vi "main_FC.vi"() -> ()   [LabVIEW 2017]
uses:
  <vilib>/addons/control/pid/pid.llb/PID (DBL).vi
  <vilib>/addons/control/pid/NI_PID_pid.lvlib
panel:
  in  "Tab Control":enum32{"Page 1", "Page 2"}(tab)
  in  "Menu Ring":u16(ring) items=["OFF", "Automatic", "Manual"]
  out "Waveform Chart":T1(graph) caption="Response Chart"
  in  "Mode":bool=TRUE
  in  "Pause Button":bool
  in  "Reset Chart":bool
  in  "Save as Excel":bool
  in  "Save as image":bool
  in  "Block Diagram":bool
  out "FR":dbl
  out "Control Action":dbl
  in  "Flow rate setpoint":dbl=25.0
  in  "Pump":bool=TRUE
  in  "ON/OFF":bool
  in  "Exit":bool
  in  "PID gains":cluster{"Kp":dbl, "KI":dbl, "Kd":dbl}={"Kp"=1.0, "KI"=0.0, "Kd"=0.0}
  out "NI1":tag caption="NI device"
  in  "Main board":bool
  # "Flow Control Training System"
  # "Flow sensor Reading"
  # "Block Diagram of \nthe Flow rate Closed-loop Control System"
  # "Automatic Mode"
  # "ON/OFF"
  # "Automatic mode"
  # "Actuator ON/OFF"
  # "desired FR"
  # "Controller\n(PID)"
  # "Actuator\n(Pump)"
  # "System"
  # "Head (d_Pressure)"
  # "error signal"
  # "+"
  # "-"
  # "Control Action\n(0% - 100%)"
  # "actual FR"
  # "Flow rate sensor"
  # "Block Diagram of \nthe Flow rate Open-loop Control System"
  # "Manual Mode"
  # "ON/OFF"
  # "Manual mode"
  # "Actuator ON/OFF"
  # "Actuator\n(Pump)"
  # "Head (d_Pressure)"
  # "System"
  # "Signal\nConditioner"
  # "Angle"
  # "Potentiometer"
  # "Control Action\n(0% - 100%)"
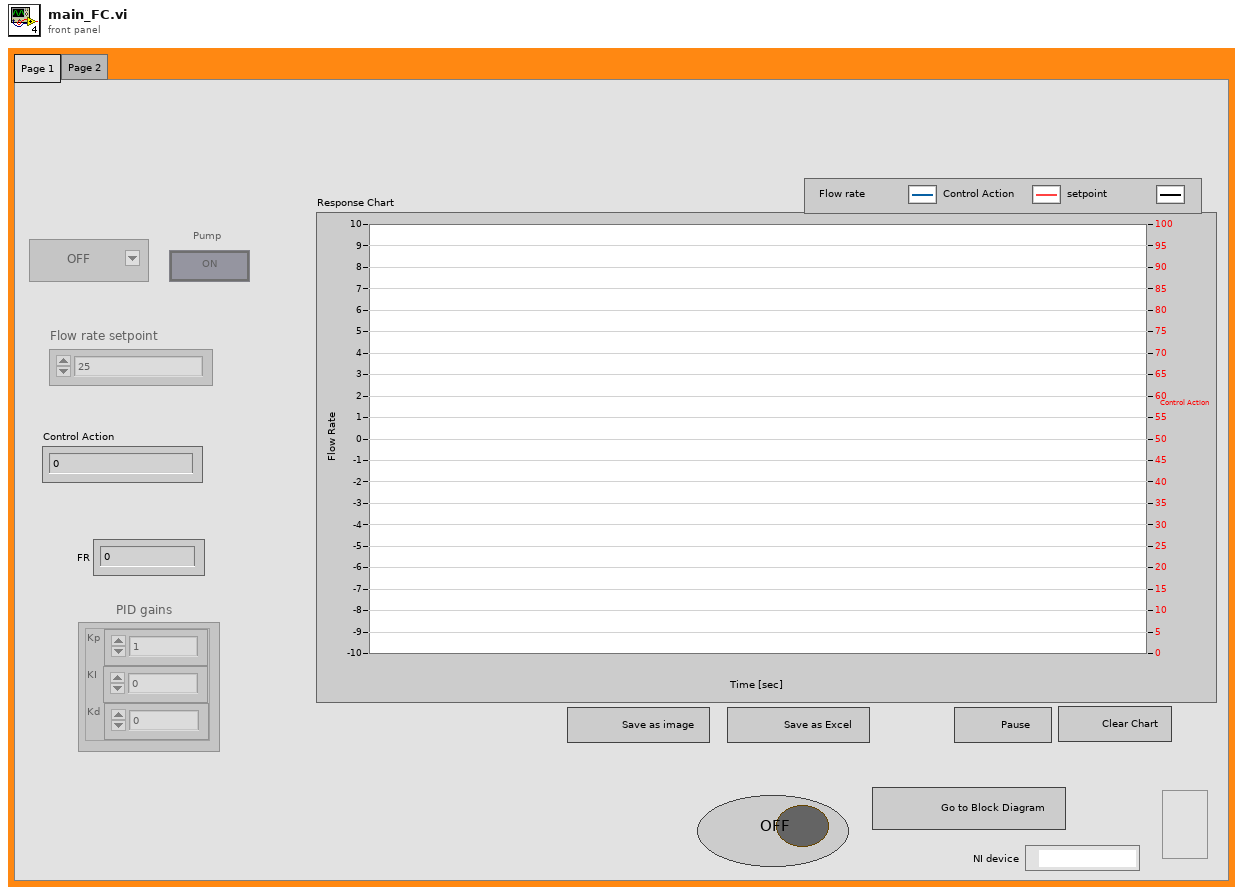
[diagram p1: front panel]
types:
  T1 = cluster{"Scalar":dbl, "f":dbl, "Flow rate setpoint":dbl}
  T2 = enum32{"Invalid", "Standard", "Closed", "Hidden", "Minimized", "Maximized"}
  T3 = enum8{"Enabled", "Disabled", "Disabled and Grayed Out"}
  T4 = cluster{"Scalar":dbl, "f":dbl, "Flow rate setpoint":dbl}[]
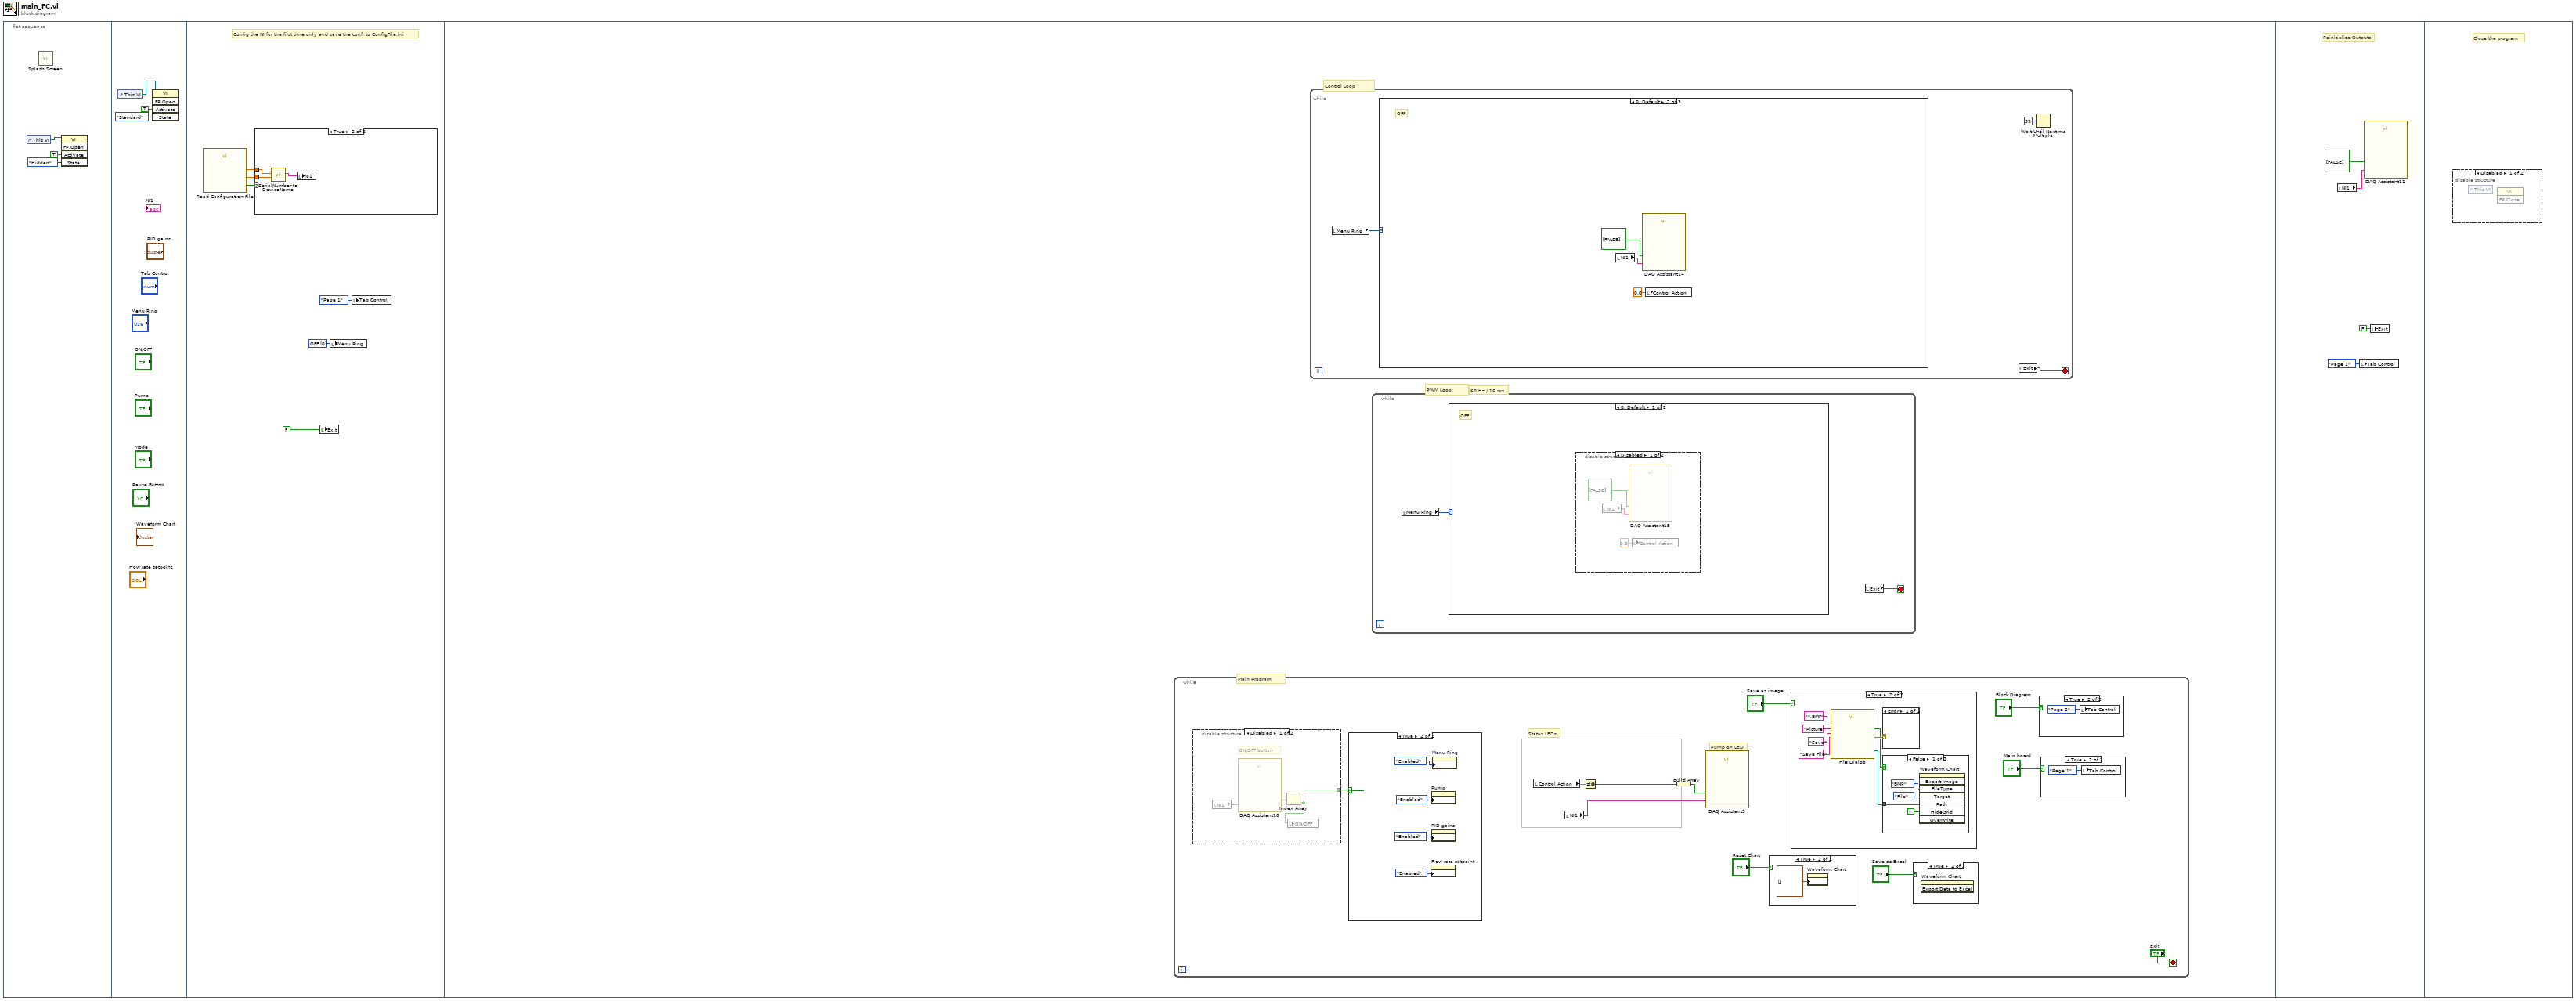
[diagram p0: block diagram]
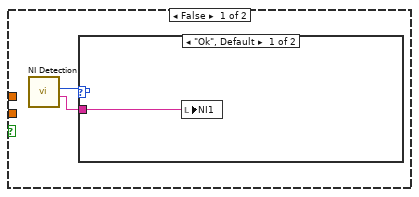
[diagram p2: hidden frame]
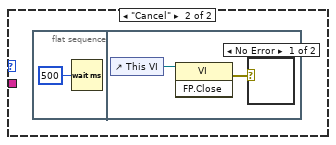
[diagram p3: hidden frame]
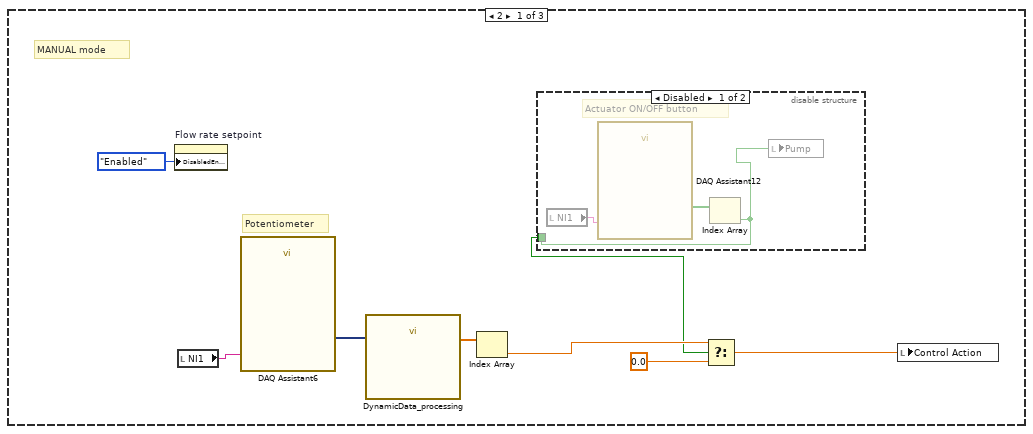
[diagram p5: hidden frame]
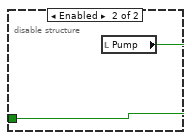
[diagram p6: hidden frame]
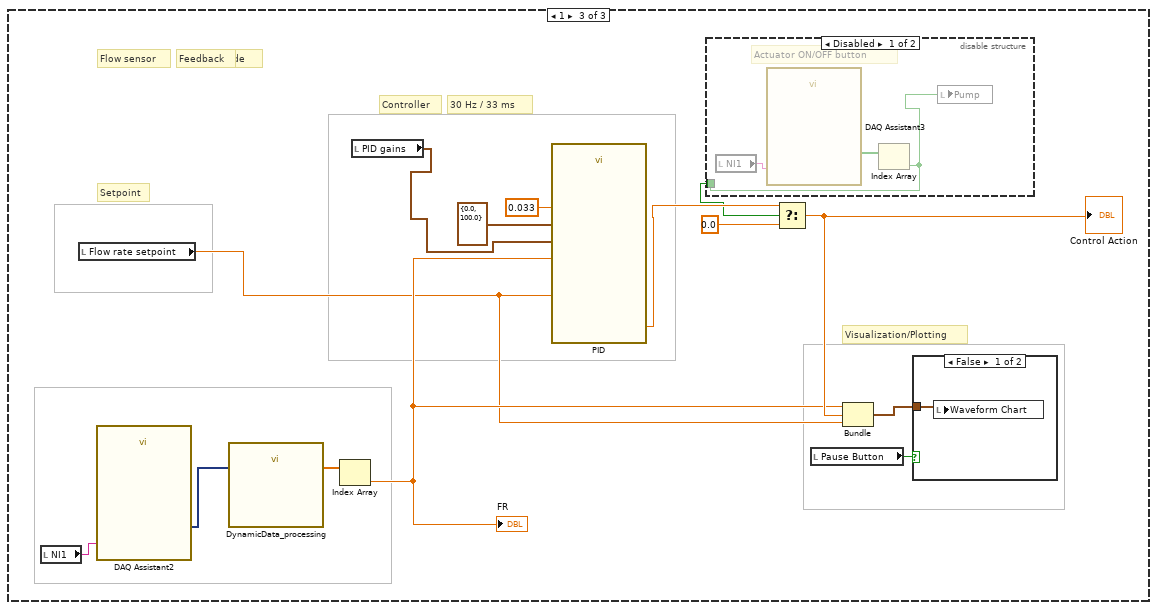
[diagram p7: hidden frame]
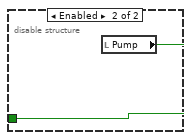
[diagram p8: hidden frame]
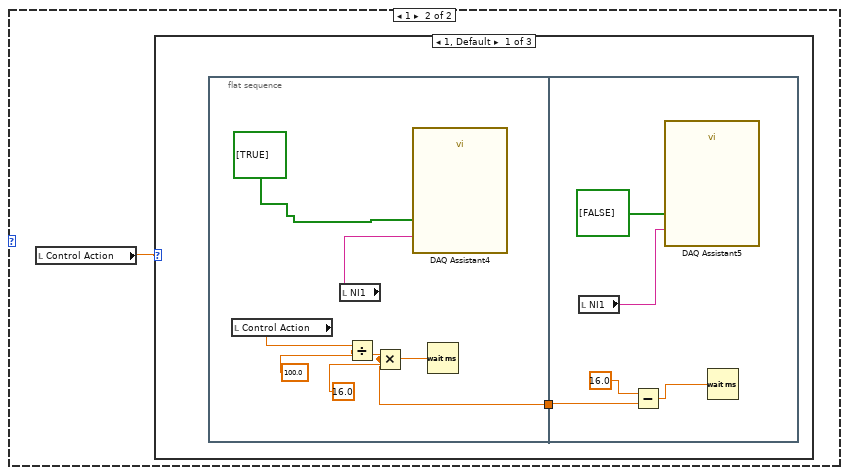
[diagram p11: hidden frame]
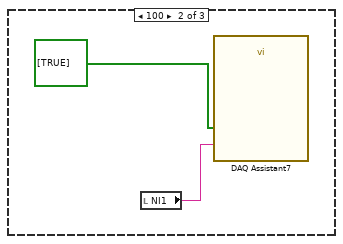
[diagram p12: hidden frame]
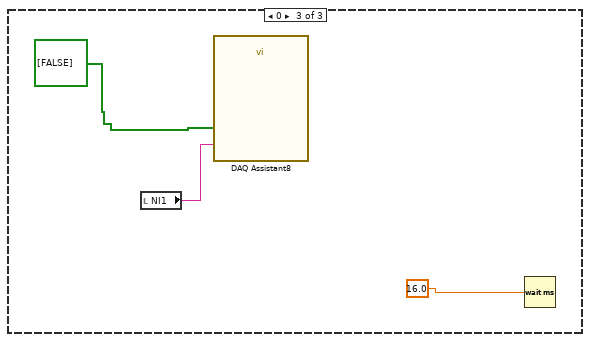
[diagram p13: hidden frame]
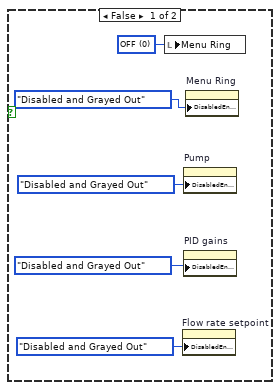
[diagram p14: hidden frame]
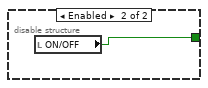
[diagram p15: hidden frame]
diagram:
  n1 = flat-sequence {
    frame #0 {
      n2 = control-ref of="This VI"() -> (w3:refnum<vi>)
      n3 = call "Splash Screen.vi"() -> ()  [unwired: 11 in, 1 out]
      n4 = invoke class="VI" method="FP.Open"(reference=w3, "Activate"=TRUE ("Activate?"), "State"=T2."Hidden") -> ()  [unwired: 2 in, 5 out]
    }
    frame #1 {
      n5 = control-ref of="This VI"() -> (w4:refnum<vi>)
      n6 = invoke class="VI" method="FP.Open"(reference=w4, "Activate"=TRUE ("Activate?"), "State"=T2."Standard") -> ()  [unwired: 2 in, 5 out]
    }
    frame #2 {
      w7 = u16 0 items=["OFF", "Automatic", "Manual"] ("Menu Ring")
      # "Config the NI for the first time only and save the conf. to ConfigFile.ini"
      n7 = call "Read Configuration File.vi"() -> ("Serial Numbers Found"=w10:bool, "NI1"=w11:dbl, "NI2"=w12:dbl)  [unwired: 13 in]
      n8 = case shown="True" w10 {
        tunnel: w11 -> [_ w21]
        tunnel: w12 -> [_ w20]
        frame False {
          n9 = call "NI Detection.vi"() -> ("NI 1"=w13:tag, "Ok/Cancel"=w14:enum16{"Ok", "Cancel"})  [unwired: 8 in, 1 out]
          n10 = case shown="\"Ok\", Default" w14 {
            tunnel: w13 -> [w15 _]
            frame "Ok", Default {
              n11 = local write "NI1"(w15) -> ()
            }
            frame "Cancel" {
              n12 = flat-sequence {
                frame #0 {
                  n13 = Wait (ms)(milliseconds to wait=u32 500) -> ()  [unwired: 1 out]
                }
                frame #1 {
                  n14 = control-ref of="This VI"() -> (w18:refnum<vi>)
                  n15 = invoke class="VI" method="FP.Close"(reference=w18) -> (error out=w17:errorcluster)  [unwired: 2 in, 2 out]
                  n16 = case shown="No Error" w17 {
                    frame No Error {
                    }
                    frame Error {
                    }
                  }
                }
              }
            }
          }
        }
        frame True {
          n17 = call "SerialNumber to DeviceName.vi"("NI2 Serial Number"=w20, "NI1 Serial Number"=w21) -> ("NI1 Device Name"=w19:tag)  [unwired: 8 in, 1 out]
          n18 = local write "NI1"(w19) -> ()
        }
      }
      n19 = local write "Exit"(FALSE ("ON / OFF program")) -> ()
      n20 = local write "Menu Ring"(w7) -> ()
      n21 = local write "Tab Control"(enum32{"Page 1", "Page 2"}."Page 1" ("Tab Control")) -> ()
    }
    frame #3 {
      # "Control Loop"
      # "60 Hz / 16 ms"
      # "PWM Loop"
      # "Main Program"
      n22 = while {
        stop <- "Exit" stop-if-true
        # "Pump on LED"
        # "Status LEDs"
        n23 = disable-structure shown="Disabled" {
          disable-tunnel: [w103 w106] -> w83
          frame Disabled {
            # "ON/OFF button"
            n24 = local read "NI1"() -> (w105:tag)
            n25 = call "DAQ Assistant10"("device name"=w105) -> ("data"=w104:bool[])  [unwired: 16 in, 2 out]
            n26 = Index Array(array=w104) -> (element=w103:bool)  [unwired: 1 in]
            n27 = local write "ON/OFF"(w103) -> ()
          }
          frame Enabled {
            n28 = local read "ON/OFF"() -> (w106:bool)
          }
        }
        n29 = case shown="True" w83 {
          frame False {
            w98 = u16 0 items=["OFF", "Automatic", "Manual"] ("Menu Ring")
            n30 = local write "Menu Ring"(w98) -> ()
            n31 = property on="Flow rate setpoint" class="DigNum (strict)"("DisabledEnum"=T3."Disabled and Grayed Out" ("Disabled")) -> ()  [unwired: 2 in, 2 out]
            n32 = property on="Pump" class="Bool (strict)"("DisabledEnum"=T3."Disabled and Grayed Out" ("Disabled")) -> ()  [unwired: 2 in, 2 out]
            n33 = property on="PID gains" class="Clust (strict)"("DisabledEnum"=T3."Disabled and Grayed Out" ("Disabled")) -> ()  [unwired: 2 in, 2 out]
            n34 = property on="Menu Ring" class="Ring (strict)"("DisabledEnum"=T3."Disabled and Grayed Out" ("Disabled")) -> ()  [unwired: 2 in, 2 out]
          }
          frame True {
            n35 = property on="Flow rate setpoint" class="DigNum (strict)"("DisabledEnum"=T3."Enabled" ("Disabled")) -> ()  [unwired: 2 in, 2 out]
            n36 = property on="Pump" class="Bool (strict)"("DisabledEnum"=T3."Enabled" ("Disabled")) -> ()  [unwired: 2 in, 2 out]
            n37 = property on="PID gains" class="Clust (strict)"("DisabledEnum"=T3."Enabled" ("Disabled")) -> ()  [unwired: 2 in, 2 out]
            n38 = property on="Menu Ring" class="Ring (strict)"("DisabledEnum"=T3."Enabled" ("Disabled")) -> ()  [unwired: 2 in, 2 out]
          }
        }
        n39 = local read "Control Action"() -> (w86:dbl)
        n40 = local read "NI1"() -> (w85:tag)
        n41 = Not Equal To 0?(x=w86) -> (x != 0?=w87:bool)
        n42 = Build Array(w87) -> (w88:bool[])
        n43 = call "DAQ Assistant9"("data"=w88, "device name"=w85) -> ()  [unwired: 16 in, 2 out]
        n44 = case shown="True" "Reset Chart" {
          frame False {
          }
          frame True {
            n45 = property on="Waveform Chart" class="WFChart (strict)"("History Data"=T4 []) -> ()  [unwired: 2 in, 2 out]
          }
        }
        n46 = case shown="True" "Save as image" {
          frame False {
          }
          frame True {
            n47 = call "File Dialog"("prompt"="Save File", "button label"="Save", "pattern (all files)"="*.BMP", "pattern label"="Picture") -> ("selected path"=w108:path, "cancelled"=w107:bool, "error out"=w109:errorcluster)  [unwired: 8 in, 1 out]
            n48 = case shown="Error" w109 {
              frame No Error {
              }
              frame Error {
              }
            }
            n49 = case shown="False" w107 {
              tunnel: w108 -> [w115 _]
              frame False {
                n50 = invoke on="Waveform Chart" class="WFChart (strict)" method="Export Image"("FileType"=enum32{"BMP", "EPS", "EMF", "PICT"}."BMP" ("File Type"), "Target"=enum32{"File", "Clipboard"}."File", "Path"=w115, "HideGrid"=TRUE ("Hide Grid")) -> ()  [unwired: 4 in, 8 out]
              }
              frame True {
              }
            }
          }
        }
        n51 = case shown="True" "Save as Excel" {
          frame False {
          }
          frame True {
            n52 = invoke on="Waveform Chart" class="WFChart (strict)" method="Export Data to Excel"() -> ()  [unwired: 3 in, 3 out]
          }
        }
        n53 = case shown="True" "Block Diagram" {
          frame False {
          }
          frame True {
            n54 = local write "Tab Control"(enum32{"Page 1", "Page 2"}."Page 2" ("Tab Control")) -> ()
          }
        }
        n55 = case shown="True" "Main board" {
          frame False {
          }
          frame True {
            n56 = local write "Tab Control"(enum32{"Page 1", "Page 2"}."Page 1" ("Tab Control")) -> ()
          }
        }
      }
      n57 = while {
        stop <- w22 stop-if-true
        n58 = local read "Menu Ring"() -> (w23:u16)
        n59 = case shown="0, Default" w23 {
          frame 2 {
            # "MANUAL mode"
            # "Potentiometer"
            n60 = property on="Flow rate setpoint" class="DigNum (strict)"("DisabledEnum"=T3."Enabled" ("Disabled")) -> ()  [unwired: 2 in, 2 out]
            n61 = local read "NI1"() -> (w32:tag)
            n62 = call "DAQ Assistant6"("device name"=w32) -> ("data"=w30:dynamicdata)  [unwired: 16 in, 2 out]
            n63 = call "DynamicData_processing.vi"("data"=w30) -> ("DATA"=w31:dbl[])
            n64 = Index Array(array=w31) -> (element=w29:dbl)  [unwired: 1 in]
            n65 = disable-structure shown="Disabled" {
              disable-tunnel: [w34 w36] -> w27
              frame Disabled {
                # "Actuator ON/OFF button"
                n66 = local read "NI1"() -> (w33:tag)
                n67 = call "DAQ Assistant12"("device name"=w33) -> ("data"=w35:bool[])  [unwired: 16 in, 2 out]
                n68 = Index Array(array=w35) -> (element=w34:bool)  [unwired: 1 in]
                n69 = local write "Pump"(w34) -> ()
              }
              frame Enabled {
                n70 = local read "Pump"() -> (w36:bool)
              }
            }
            n71 = Select(t=w29, s=w27, f=0.0) -> (s? t:f=w28:dbl)
            n72 = local write "Control Action"(w28) -> ()
          }
          frame 0, Default {
            # "OFF"
            n73 = local read "NI1"() -> (w39:tag)
            n74 = call "DAQ Assistant14"("data"=bool[] [FALSE], "device name"=w39) -> ()  [unwired: 16 in, 2 out]
            n75 = local write "Control Action"(0.0 ("Control Action")) -> ()
          }
          frame 1 {
            # "AUTO mode"
            # "Setpoint"
            # "Visualization/Plotting"
            # "Controller"
            # "Feedback"
            # "30 Hz / 33 ms"
            # "Flow sensor"
            n76 = local read "NI1"() -> (w47:tag)
            n77 = local read "Flow rate setpoint"() -> (w40:dbl)
            n78 = call "DAQ Assistant2"("device name"=w47) -> ("data"=w53:dynamicdata)  [unwired: 16 in, 2 out]
            n79 = call "DynamicData_processing.vi"("data"=w53) -> ("DATA"=w52:dbl[])
            n80 = Index Array(array=w52) -> (element=w43:dbl)  [unwired: 1 in]
            "FR" <- w43
            n81 = local read "PID gains"() -> (w41:cluster{"Kp":dbl, "KI":dbl, "Kd":dbl})
            n82 = call-poly <vilib>:"PID.vi"("output range"=cluster{"output high":dbl, "output low":dbl} {"output high"=0.0, "output low"=100.0}, "dt (s)"=0.033, "PID gains"=w41, "process variable"=w43, "setpoint"=w40) -> ("output"=w50:dbl)  [unwired: 5 in, 1 out]
            n83 = disable-structure shown="Disabled" {
              disable-tunnel: [w55 w57] -> w44
              frame Disabled {
                # "Actuator ON/OFF button"
                n84 = local read "NI1"() -> (w54:tag)
                n85 = call "DAQ Assistant3"("device name"=w54) -> ("data"=w56:bool[])  [unwired: 16 in, 2 out]
                n86 = Index Array(array=w56) -> (element=w55:bool)  [unwired: 1 in]
                n87 = local write "Pump"(w55) -> ()
              }
              frame Enabled {
                n88 = local read "Pump"() -> (w57:bool)
              }
            }
            n89 = Select(t=w50, s=w44, f=0.0) -> (s? t:f=w45:dbl)
            "Control Action" <- w45
            n90 = local read "Pause Button"() -> (w42:bool)
            n91 = Bundle("Scalar"=w43, "f"=w45, "Flow rate setpoint"=w40) -> (w48:T1)  [unwired: 1 in]
            n92 = case shown="False" w42 {
              tunnel: w48 -> [w58 _]
              frame False {
                n93 = local write "Waveform Chart"(w58) -> ()
              }
              frame True {
              }
            }
          }
        }
        n94 = local read "Exit"() -> (w22:bool)
        n95 = Wait Until Next ms Multiple(millisecond multiple=u32 33) -> ()  [unwired: 1 out]
      }
      n96 = while {
        stop <- w59 stop-if-true
        n97 = local read "Menu Ring"() -> (w60:u16)
        n98 = case shown="0, Default" w60 {
          frame 0, Default {
            # "OFF"
            n99 = disable-structure shown="Disabled" {
              frame Disabled {
                n100 = local read "NI1"() -> (w61:tag)
                n101 = call "DAQ Assistant15"("data"=bool[] [FALSE], "device name"=w61) -> ()  [unwired: 16 in, 2 out]
                n102 = local write "Control Action"(0.0 ("Control Action")) -> ()
              }
              frame Enabled {
              }
            }
          }
          frame 1 {
            n103 = local read "Control Action"() -> (w64:dbl)
            n104 = case shown="1, Default" w64 {
              frame 1, Default {
                n105 = flat-sequence {
                  tunnel: [w69] -> w65
                  tunnel: w65 -> [w77]
                  frame #0 {
                    n106 = local read "Control Action"() -> (w66:dbl)
                    n107 = local read "NI1"() -> (w68:tag)
                    n108 = Divide(x=w66, y=100.0) -> (x/y=w71:dbl)
                    n109 = Multiply(x=w71, y=16.0) -> (x*y=w69:dbl)
                    n110 = call "DAQ Assistant4"("data"=bool[] [TRUE], "device name"=w68) -> ()  [unwired: 16 in, 2 out]
                    n111 = Wait (ms)(milliseconds to wait=w69) -> ()  [unwired: 1 out]
                  }
                  frame #1 {
                    n112 = local read "NI1"() -> (w74:tag)
                    n113 = Subtract(x=16.0 ("y"), y=w77) -> (x-y=w75:dbl)
                    n114 = call "DAQ Assistant5"("data"=bool[] [FALSE], "device name"=w74) -> ()  [unwired: 16 in, 2 out]
                    n115 = Wait (ms)(milliseconds to wait=w75) -> ()  [unwired: 1 out]
                  }
                }
              }
              frame 100 {
                n116 = local read "NI1"() -> (w79:tag)
                n117 = call "DAQ Assistant7"("data"=bool[] [TRUE], "device name"=w79) -> ()  [unwired: 16 in, 2 out]
              }
              frame 0 {
                n118 = local read "NI1"() -> (w82:tag)
                n119 = call "DAQ Assistant8"("data"=bool[] [FALSE], "device name"=w82) -> ()  [unwired: 16 in, 2 out]
                n120 = Wait (ms)(milliseconds to wait=16.0 ("y")) -> ()  [unwired: 1 out]
              }
            }
          }
        }
        n121 = local read "Exit"() -> (w59:bool)
      }
    }
    frame #4 {
      # "Reinitialize Outputs"
      n122 = local read "NI1"() -> (w123:tag)
      n123 = local write "Tab Control"(enum32{"Page 1", "Page 2"}."Page 1" ("Tab Control")) -> ()
      n124 = call "DAQ Assistant11"("data"=bool[] [FALSE], "device name"=w123) -> ()  [unwired: 16 in, 2 out]
      n125 = local write "Exit"(FALSE ("Exit")) -> ()
    }
    frame #5 {
      # "Close the program"
      n126 = disable-structure shown="Disabled" {
        frame Disabled {
          n127 = control-ref of="This VI"() -> (w125:refnum<vi>)
          n128 = invoke class="VI" method="FP.Close"(reference=w125) -> ()  [unwired: 2 in, 3 out]
        }
        frame Enabled {
        }
      }
    }
  }
